vi "Initialize Log.vi"(8 "error in (no error)":errorcluster, 11 "Log Path":path=path "C:/Logs") -> (0 "error out":errorcluster, 3 "refnum out":refnum<file>)   [LabVIEW 2019, in "GUI.lvlib"]
doc: "EnQ:\nMACRO:Initialize"
uses:
  GUI.lvlib
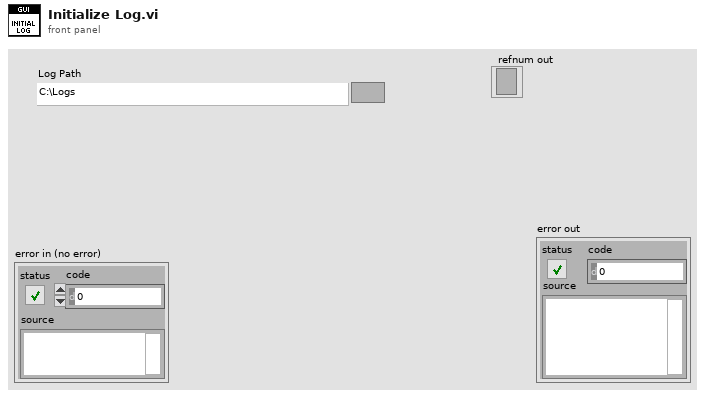
[diagram p1: front panel]
types:
  T1 = enum16{"open", "replace", "create", "open or create", "replace or create", "replace or create with confirmation"}
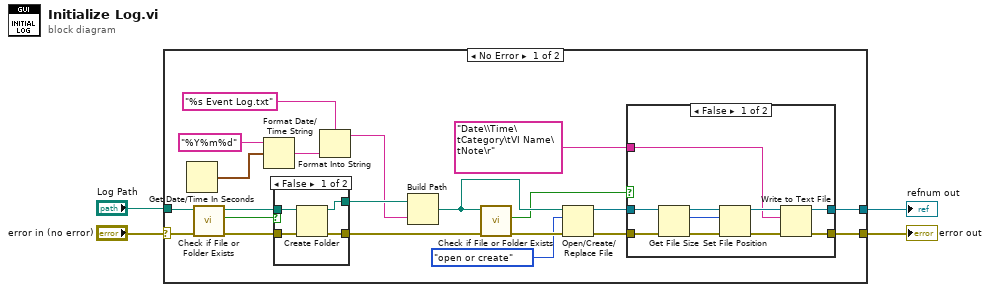
[diagram p0: block diagram]
diagram:
  n1 = case shown="No Error" "error in (no error)" {
    selector: "error in (no error)" -> [w10 w44]
    tunnel: [w9 w44] -> w3
    tunnel: "Log Path" -> [w8 _]
    tunnel: [w5 _] -> w1
    frame No Error {
      n2 = Get Date/Time In Seconds() -> (seconds since 1Jan1904=w20:timestamp)
      n3 = call <vilib>:"Check if File or Folder Exists.vi"("error in (no error)"=w10, "path"=w8) -> ("error out"=w21:errorcluster, "file or folder exists?"=w24:bool, "dup path"=w23:path)  [unwired: 7 in]
      n4 = Format Date/Time String(time format string (%c)="%Y%m%d", seconds (now)=w20) -> (date/time string=w19:string)  [unwired: 1 in]
      n5 = case shown="False" w24 {
        tunnel: w23 -> [w41 w43]
        tunnel: [w40 w43] -> w22
        tunnel: w21 -> [w39 w42]
        tunnel: [w38 w42] -> w14
        frame False {
          n6 = Create Folder(path (use dialog)=w41, error in=w39) -> (created path=w40:path, error out=w38:errorcluster)  [unwired: 1 in, 1 out]
        }
        frame True {
        }
      }
      n7 = Format Into String(format string="%s Event Log.txt" ("name or relative path"), w19) -> (resulting string=w18:string)  [unwired: 2 in, 1 out]
      n8 = Build Path(base path=w22, name or relative path=w18) -> (appended path=w16:path)
      n9 = call <vilib>:"Check if File or Folder Exists.vi"("error in (no error)"=w14, "path"=w16) -> ("error out"=w13:errorcluster, "file or folder exists?"=w15:bool)  [unwired: 7 in, 1 out]
      n10 = Open/Create/Replace File(file path (use dialog)=w16, error in=w13, operation (0:open)=T1."open or create") -> (refnum out=w17:refnum<file>, error out=w25:errorcluster)  [unwired: 3 in, 1 out]
      n11 = case shown="False" w15 {
        tunnel: w25 -> [w35 w36]
        tunnel: [w34 w36] -> w9
        tunnel: w17 -> [w31 w37]
        tunnel: [w33 w37] -> w5
        tunnel: "Date\\Time\tCategory\tVI Name\tNote\r" ("text") -> [w26 _]
        frame False {
          n12 = Get File Size(file=w31, error in=w35) -> (refnum out=w29:refnum<file>, size (in bytes)=w27:i64, 0:w32:errorcluster)
          n13 = Set File Position(offset (in bytes) (0)=w27, refnum=w29, error in=w32) -> (refnum out=w28:refnum<file>, error out=w30:errorcluster)  [unwired: 1 in]
          n14 = Write to Text File(file (use dialog)=w28, text=w26, error in=w30) -> (refnum out=w33:refnum<file>, error out=w34:errorcluster)  [unwired: 1 in, 1 out]
        }
        frame True {
        }
      }
    }
    frame Error {
    }
  }
  "error out" <- w3
  "refnum out" <- w1
